vi "xijk_combined_single_file_main.vi"(8 "error in (no error)":errorcluster, 9 "channel":string, 10 "element":string="#EX", 11 "file path in":path) -> (0 "error out":errorcluster, 3 "file path out":path, 4 "cube file present?":bool)   [LabVIEW 2010, in "xijk_combined_file.lvlib"]
uses:
  xijk_combined_file.lvlib
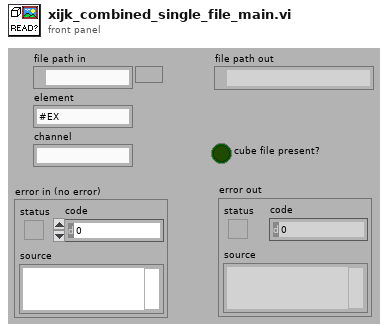
[diagram p1: front panel]
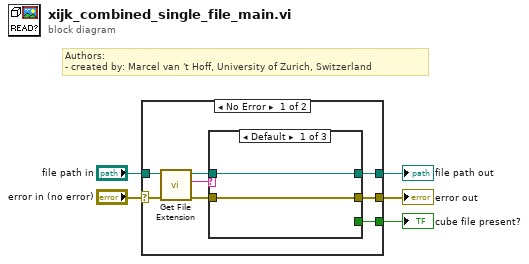
[diagram p0: block diagram]
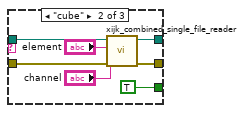
[diagram p2: hidden frame]
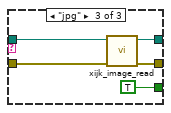
[diagram p3: hidden frame]
diagram:
  # "Authors: \n- created by: Marcel van 't Hoff, University of Zurich, Switzerland"
  n1 = case shown="No Error" "error in (no error)" {
    selector: "error in (no error)" -> [w10 w28]
    tunnel: [w12 w27] -> w5
    tunnel: "file path in" -> [w11 w27]
    tunnel: [w8 w28] -> w3
    tunnel: [w6 _] -> w1
    frame No Error {
      n2 = call <vilib>:"Get File Extension.vi"("error in (no error)"=w10, "file"=w11) -> ("error out"=w9:errorcluster, "lowercase file extension"=w7:string)  [unwired: 6 in, 2 out]
      n3 = case shown="Default" w7 {
        tunnel: w11 -> [w14 w21 w26]
        tunnel: [w14 w20 w25] -> w12
        tunnel: w9 -> [w13 w17 w24]
        tunnel: [w13 w16 w23] -> w8
        tunnel: [_ TRUE TRUE] -> w6
        frame Default {
        }
        frame "cube" {
          n4 = call "xijk_combined_single_file_reader.vi"("error in (no error)"=w17, "channel"="channel", "element"="element", "file path input"=w21) -> ("error out"=w16:errorcluster, "file path out"=w20:path)  [unwired: 6 in]
        }
        frame "jpg" {
          n5 = call "xijk_image_read.vi"("error in (no error)"=w24, "path in"=w26) -> ("error out"=w23:errorcluster, "path out"=w25:path)  [unwired: 8 in]
        }
      }
    }
    frame Error {
    }
  }
  "file path out" <- w5
  "error out" <- w3
  "cube file present?" <- w1
